vi "MoveArmForTime.vi"() -> ()   [LabVIEW 2017]
panel:
  in  "NoWait":bool
  in  "Time":dbl
  in  "Speed":dbl
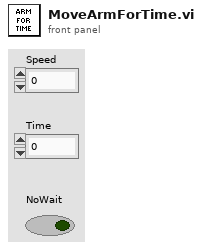
[diagram p1: front panel]
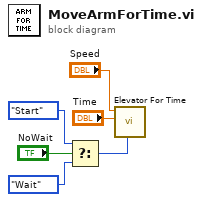
[diagram p0: block diagram]
diagram:
  n1 = Select(t=enum16{"Start", "Wait"}."Start" ("Synchronization"), s="NoWait", f=enum16{"Start", "Wait"}."Wait" ("Synchronization")) -> (s? t:f=w1:enum16{"Start", "Wait"})
  n2 = call "Elevator For Time.vi"("Synchronization"=w1, "Duration (s)"="Time", "Setpoint"="Speed") -> ()  [unwired: 8 in, 1 out]
